vi "Start Sync.vi"(8 "error in (no error)":errorcluster, 11 "gRPC Server in":refnum<class "GreeterService.lvclass">) -> (0 "error out":errorcluster, 3 "gRPC Server out":refnum<class "GreeterService.lvclass">)   [LabVIEW 2019, in "Generated_server.lvlib" / "GreeterService.lvclass"]
uses:
  GreeterService.lvclass
  GreeterService.lvclass/GreeterService.ctl
  RPC Messages/Response.ctl
  RPC Messages/Response_response_oneof/Response_response_oneof.lvclass
  RPC Messages/Request_request_oneof/Request_request_oneof.lvclass/Request_request_oneof.ctl
  RPC Messages/Response_response_oneof/Response_response_oneof.lvclass/Response_response_oneof.ctl
  Generated_server.lvlib
  RPC Messages/Request_request_oneof/Request_request_oneof.lvclass
  <vilib>/gRPC/LabVIEW gRPC Library/grpc-lvsupport-release.lvlib
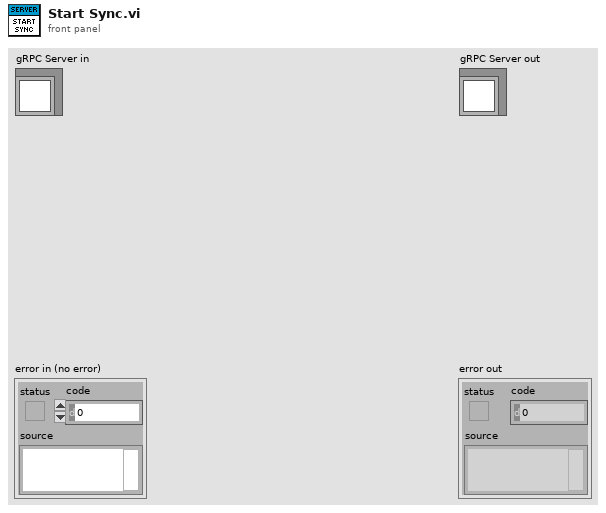
[diagram p1: front panel]
types:
  T1 = typedef "Generated_server.lvlib/Response.ctl" = cluster{"new_age":i32, "Response_response_oneof":refnum<class "Response_response_oneof.lvclass">}
  T2 = typedef "Generated_server.lvlib/GreeterService.lvclass/Server Internal UEs.ctl" = cluster{"GreeterService UnaryMethod Internal UE":refnum<user-event>, "GreeterService ServerStreamingMethod Internal UE":refnum<user-event>, "GreeterService ClientStreamingMethod Internal UE":refnum<user-event>, "GreeterService BidirectionalStreamingMethod Internal UE":refnum<user-event>}
  T3 = typedef "Generated_server.lvlib/GreeterService.lvclass/Server gRPC UEs.ctl" = cluster{"GreeterService UnaryMethod gRPC UE":refnum<user-event>, "GreeterService ServerStreamingMethod gRPC UE":refnum<user-event>, "GreeterService ClientStreamingMethod gRPC UE":refnum<user-event>, "GreeterService BidirectionalStreamingMethod gRPC UE":refnum<user-event>}
  T4 = typedef "grpc-lvsupport-release.lvlib/grpcId.ctl" = u64
  T5 = typedef "Generated_server.lvlib/Request.ctl" = cluster{"age":i32, "Request_request_oneof":refnum<class "Request_request_oneof.lvclass">}
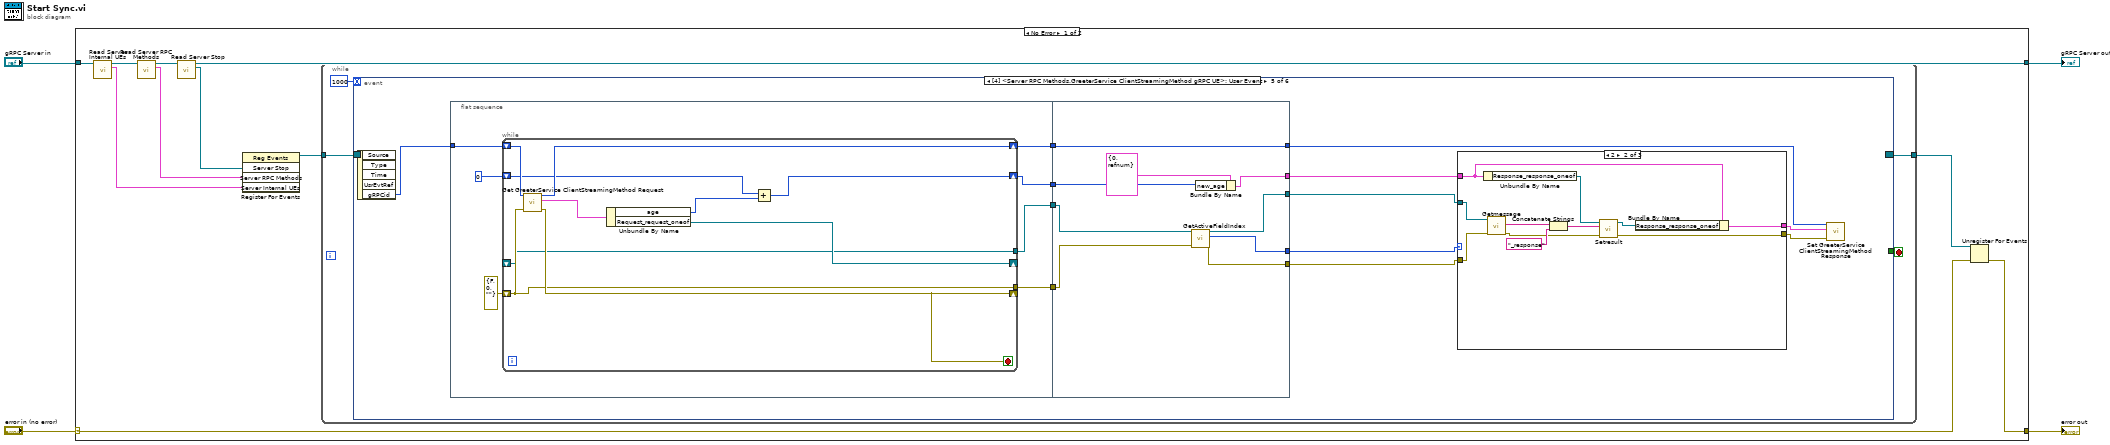
[diagram p0: block diagram]
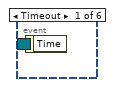
[diagram p2: hidden frame]
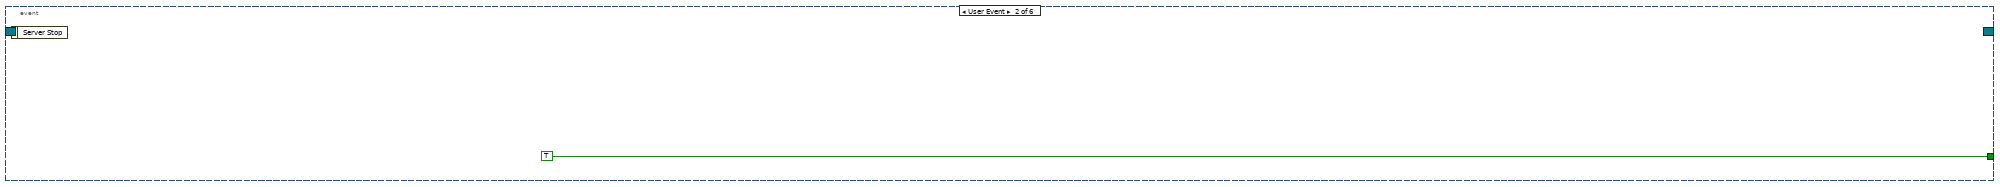
[diagram p3: hidden frame]
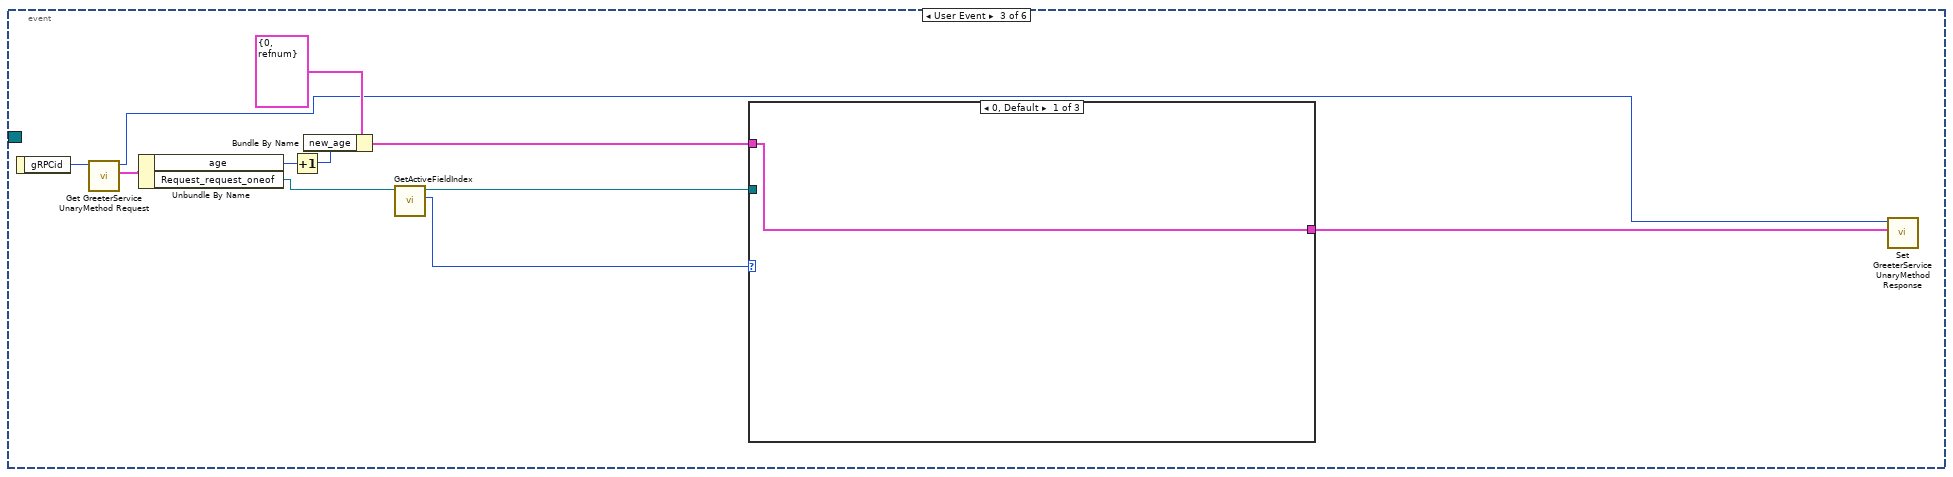
[diagram p4: hidden frame]
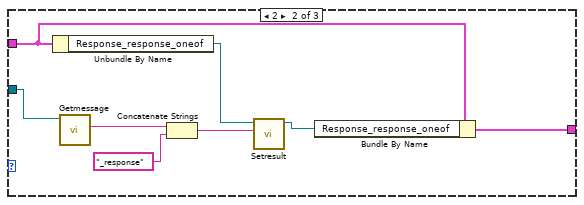
[diagram p5: hidden frame]
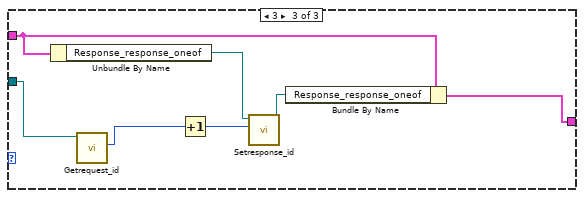
[diagram p6: hidden frame]
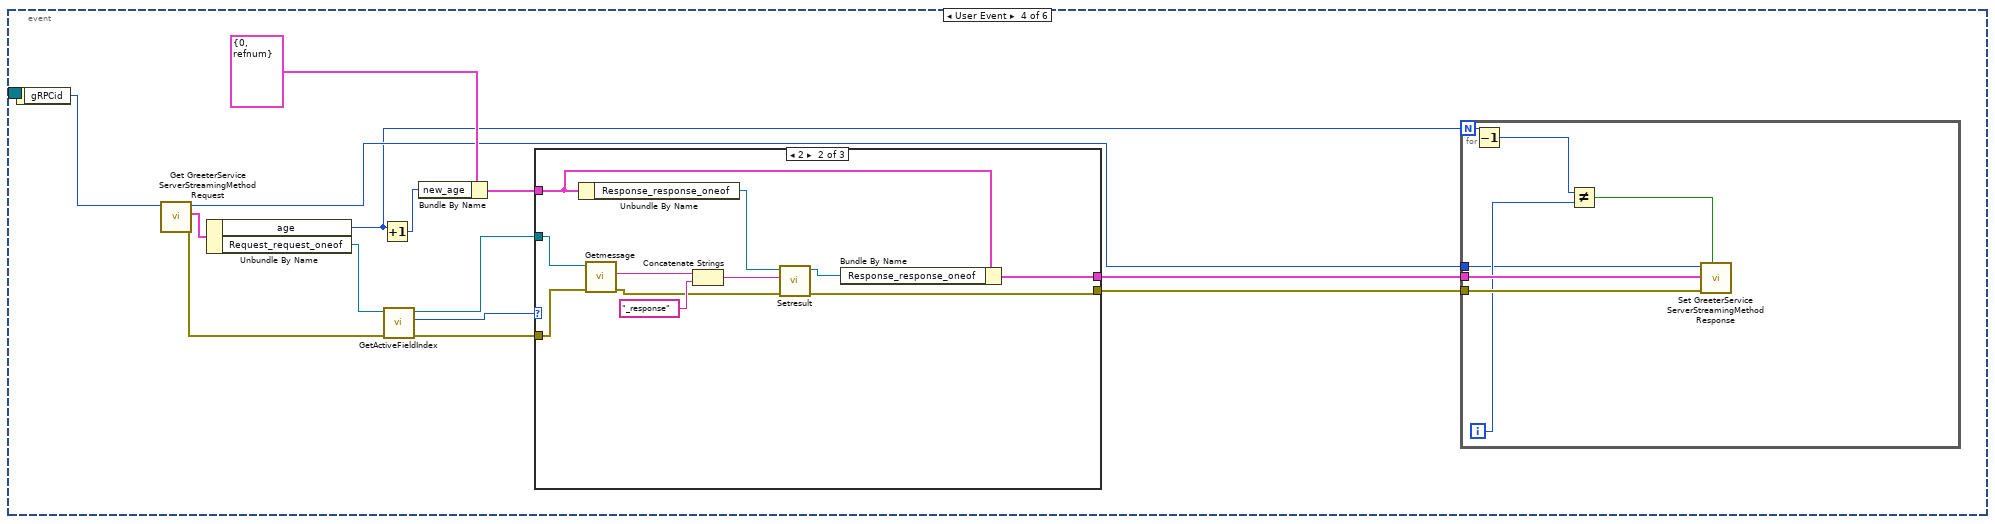
[diagram p7: hidden frame]
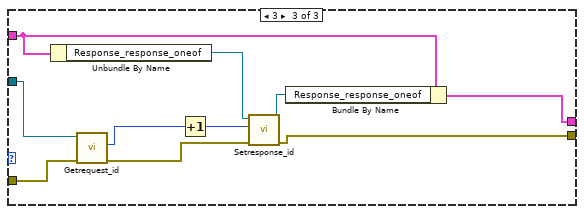
[diagram p9: hidden frame]
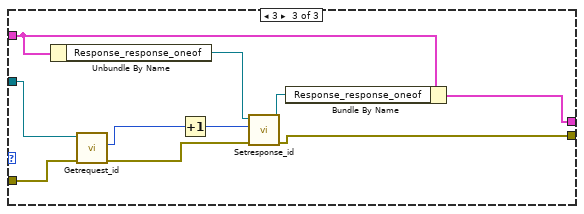
[diagram p11: hidden frame]
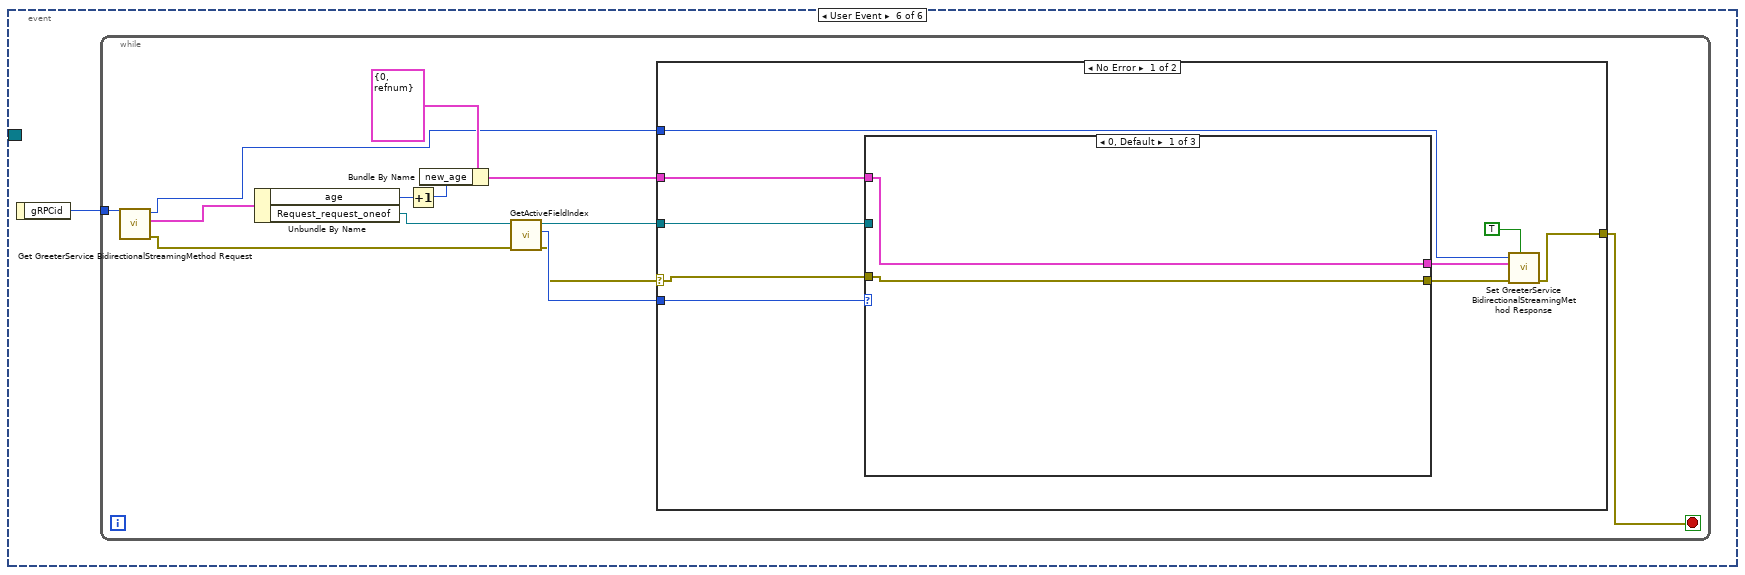
[diagram p12: hidden frame]
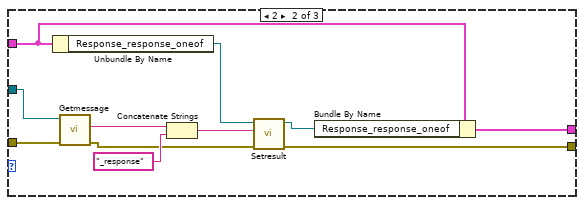
[diagram p13: hidden frame]
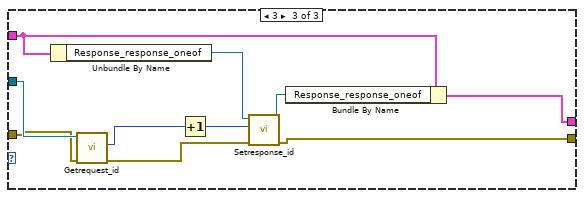
[diagram p14: hidden frame]
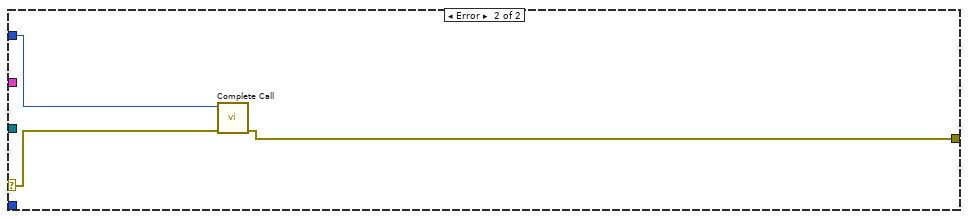
[diagram p15: hidden frame]
diagram:
  n1 = case shown="No Error" "error in (no error)" {
    selector: "error in (no error)" -> [w9 w203]
    tunnel: [w8 w203] -> w3
    tunnel: [w6 w202] -> w1
    tunnel: "gRPC Server in" -> [w15 w202]
    frame No Error {
      n2 = call "Read Server Internal UEs.vi"("SignalGeneratorService in"=w15) -> ("Server Internal UEs"=w13:T2, "SignalGeneratorService out"=w14:refnum<class "GreeterService.lvclass">)  [unwired: 8 in, 1 out]
      n3 = call "Read Server RPC Methods.vi"("SignalGeneratorService in"=w14) -> ("Server RPC Methods"=w7:T3, "SignalGeneratorService out"=w12:refnum<class "GreeterService.lvclass">)  [unwired: 8 in, 1 out]
      n4 = call-dynamic "Read Server Stop.vi"("iService in"=w12) -> ("Server Stop"=w5:refnum<user-event>, "iService out"=w6:refnum<class "GreeterService.lvclass">)  [unwired: 8 in, 1 out]
      n5 = register-events(w5, w7, w13) -> (reference out=w11:refnum<event-registration>)  [unwired: 2 in, 1 out]
      n6 = while {
        tunnel: w11 -> [w19]
        tunnel: [w17] -> w10
        stop <- w18 stop-if-true
        n7 = event "RPC Methods Event Structure" shown="[4] <Server RPC Methods.GreeterService ClientStreamingMethod gRPC UE>: User Event" {
          selector: w19 -> [_ _ _ _ _ _]
          dyn-events: [_ _ _ _ _ _] -> w17
          timeout: 1000 -> [_ _ _ _ _ _]
          tunnel: [_ TRUE _ _ _ _] -> w18
          event Timeout {
            n8 = event-data() -> ()  [unwired: 1 in, 1 out]
          }
          event User Event {
            n9 = event-data() -> ()  [unwired: 1 in, 1 out]
          }
          event User Event {
            n10 = event-data() -> ("gRPCid"=w31:T4)  [unwired: 1 in]
            n11 = call "Get GreeterService UnaryMethod Request.vi"("gRPCid"=w31) -> ("Message Data"=w30:T5, "gRPCid out"=w21:T4)  [unwired: 8 in, 1 out]
            n12 = Unbundle By Name(w30) -> ("age"=w27:i32, "Request_request_oneof"=w26:refnum<class "Request_request_oneof.lvclass">)
            n13 = Increment(x=w27) -> (x+1=w28:i32)
            n14 = Bundle By Name(cluster=T1 {"new_age"=0, "Response_response_oneof"=refnum} ("Response"), "new_age"=w28) -> (w23:T1)
            n15 = call "GetActiveFieldIndex.vi"("OneOfTemplate in"=w26) -> ("Active Field Index"=w25:i32, "OneOfTemplate out"=w24:refnum<class "Request_request_oneof.lvclass">)  [unwired: 8 in, 1 out]
            n16 = case shown="0, Default" w25 {
              tunnel: w24 -> [_ w40 w47]
              tunnel: w23 -> [w32 w35 w43]
              tunnel: [w32 w33 w41] -> w22
              frame 0, Default {
              }
              frame 2 {
                n17 = Unbundle By Name(w35) -> ("Response_response_oneof"=w36:refnum<class "Response_response_oneof.lvclass">)
                n18 = call "Getmessage.vi"("OneOfTemplate in"=w40) -> ("Get_Val"=w39:string)  [unwired: 8 in, 2 out]
                n19 = Concatenate Strings(w39, "_response") -> (w37:string)
                n20 = call "Setresult.vi"("Set_Val"=w37, "OneOfTemplate in"=w36) -> ("OneOfTemplate out"=w34:refnum<class "Response_response_oneof.lvclass">)  [unwired: 8 in, 1 out]
                n21 = Bundle By Name(cluster=w35, "Response_response_oneof"=w34) -> (w33:T1)
              }
              frame 3 {
                n22 = Unbundle By Name(w43) -> ("Response_response_oneof"=w44:refnum<class "Response_response_oneof.lvclass">)
                n23 = call "Getrequest_id.vi"("OneOfTemplate in"=w47) -> ("Get_Val"=w46:i32)  [unwired: 8 in, 2 out]
                n24 = Increment(x=w46) -> (x+1=w45:i32)
                n25 = call "Setresponse_id.vi"("Set_Val"=w45, "OneOfTemplate in"=w44) -> ("OneOfTemplate out"=w42:refnum<class "Response_response_oneof.lvclass">)  [unwired: 8 in, 1 out]
                n26 = Bundle By Name(cluster=w43, "Response_response_oneof"=w42) -> (w41:T1)
              }
            }
            n27 = call "Set GreeterService UnaryMethod Response.vi"("Message Data"=w22, "gRPCid in"=w21) -> ()  [unwired: 9 in, 1 out]
          }
          event User Event {
            n28 = event-data() -> ("gRPCid"=w61:T4)  [unwired: 1 in]
            n29 = call "Get GreeterService ServerStreamingMethod Request.vi"("gRPCid"=w61) -> ("error out"=w52:errorcluster, "Message Data"=w60:T5, "gRPCid out"=w49:T4)  [unwired: 8 in]
            n30 = Unbundle By Name(w60) -> ("age"=w48:i32, "Request_request_oneof"=w57:refnum<class "Request_request_oneof.lvclass">)
            n31 = Increment(x=w48) -> (x+1=w54:i32)
            n32 = call "GetActiveFieldIndex.vi"("error in (no error)"=w52, "OneOfTemplate in"=w57) -> ("error out"=w51:errorcluster, "Active Field Index"=w55:i32, "OneOfTemplate out"=w56:refnum<class "Request_request_oneof.lvclass">)  [unwired: 7 in]
            n33 = Bundle By Name(cluster=T1 {"new_age"=0, "Response_response_oneof"=refnum} ("Response"), "new_age"=w54) -> (w58:T1)
            n34 = case shown="2" w55 {
              tunnel: w56 -> [_ w74 w84]
              tunnel: w58 -> [w63 w69 w80]
              tunnel: [w63 w67 w78] -> w53
              tunnel: w51 -> [w62 w66 w77]
              tunnel: [w62 w64 w75] -> w50
              frame 0, Default {
              }
              frame 2 {
                n35 = Unbundle By Name(w69) -> ("Response_response_oneof"=w70:refnum<class "Response_response_oneof.lvclass">)
                n36 = call "Getmessage.vi"("error in (no error)"=w66, "OneOfTemplate in"=w74) -> ("error out"=w65:errorcluster, "Get_Val"=w73:string)  [unwired: 7 in, 1 out]
                n37 = Concatenate Strings(w73, "_response") -> (w71:string)
                n38 = call "Setresult.vi"("error in (no error)"=w65, "Set_Val"=w71, "OneOfTemplate in"=w70) -> ("error out"=w64:errorcluster, "OneOfTemplate out"=w68:refnum<class "Response_response_oneof.lvclass">)  [unwired: 7 in]
                n39 = Bundle By Name(cluster=w69, "Response_response_oneof"=w68) -> (w67:T1)
              }
              frame 3 {
                n40 = Unbundle By Name(w80) -> ("Response_response_oneof"=w81:refnum<class "Response_response_oneof.lvclass">)
                n41 = call "Getrequest_id.vi"("error in (no error)"=w77, "OneOfTemplate in"=w84) -> ("error out"=w76:errorcluster, "Get_Val"=w83:i32)  [unwired: 7 in, 1 out]
                n42 = Increment(x=w83) -> (x+1=w82:i32)
                n43 = call "Setresponse_id.vi"("error in (no error)"=w76, "Set_Val"=w82, "OneOfTemplate in"=w81) -> ("error out"=w75:errorcluster, "OneOfTemplate out"=w79:refnum<class "Response_response_oneof.lvclass">)  [unwired: 7 in]
                n44 = Bundle By Name(cluster=w80, "Response_response_oneof"=w79) -> (w78:T1)
              }
            }
            n45 = for {
              N: w48 -> [w86]
              tunnel: w53 -> [w91]
              tunnel: w50 -> [w90]
              tunnel: w49 -> [w87]
              i -> [w89]
              n46 = Decrement(x=w86) -> (x-1=w85:i32)
              n47 = Not Equal?(x=w85, y=w89) -> (x != y?=w88:bool)
              n48 = call "Set GreeterService ServerStreamingMethod Response.vi"("Streaming? (F)"=w88, "error in (no error)"=w90, "Message Data"=w91, "gRPCid in"=w87) -> ()  [unwired: 7 in, 1 out]
            }
          }
          event User Event {
            n49 = event-data() -> ("gRPCid"=w103:T4)  [unwired: 1 in, 4 out]
            n50 = flat-sequence {
              tunnel: w103 -> [w110]
              tunnel: [w108] -> w100
              tunnel: [w107] -> w99
              tunnel: [w106] -> w98
              tunnel: [w105] -> w97
              tunnel: [w129] -> w92
              tunnel: w100 -> [w125]
              tunnel: w99 -> [w129]
              tunnel: w98 -> [w128]
              tunnel: w97 -> [w127]
              tunnel: [w124] -> w96
              tunnel: [w123] -> w95
              tunnel: [w122] -> w94
              tunnel: [w121] -> w93
              frame #0 {
                n51 = while {
                  shift-right: [w115] -> w108
                  shift-left: 0 -> [w116]
                  shift-right: [w114] -> _
                  shift-left: _ -> [w111]
                  shift-right: [w118] -> w107
                  shift-left: w110 -> [w119]
                  shift-right: [w113] -> _
                  shift-left: errorcluster {"status"=FALSE, "code"=0, "source"=""} ("error out") -> [w112]
                  tunnel: [w112] -> w106
                  tunnel: [w111] -> w105
                  stop <- w113 stop-if-true
                  n52 = call "Get GreeterService ClientStreamingMethod Request.vi"("error in (no error)"=w112, "gRPCid"=w119) -> ("error out"=w113:errorcluster, "Message Data"=w120:T5, "gRPCid out"=w118:T4)  [unwired: 7 in]
                  n53 = Unbundle By Name(w120) -> ("age"=w117:i32, "Request_request_oneof"=w114:refnum<class "Request_request_oneof.lvclass">)
                  n54 = Add(x=w116, y=w117) -> (x+y=w115:i32)
                }
              }
              frame #1 {
                n55 = call "GetActiveFieldIndex.vi"("error in (no error)"=w128, "OneOfTemplate in"=w127) -> ("error out"=w124:errorcluster, "Active Field Index"=w123:i32, "OneOfTemplate out"=w122:refnum<class "Request_request_oneof.lvclass">)  [unwired: 7 in]
                n56 = Bundle By Name(cluster=T1 {"new_age"=0, "Response_response_oneof"=refnum} ("Response"), "new_age"=w125) -> (w121:T1)
              }
            }
            n57 = case shown="2" w95 {
              tunnel: w94 -> [_ w142 w152]
              tunnel: w93 -> [w131 w137 w148]
              tunnel: [w131 w135 w146] -> w102
              tunnel: w96 -> [w130 w134 w145]
              tunnel: [w130 w132 w143] -> w101
              frame 0, Default {
              }
              frame 2 {
                n58 = Unbundle By Name(w137) -> ("Response_response_oneof"=w138:refnum<class "Response_response_oneof.lvclass">)
                n59 = call "Getmessage.vi"("error in (no error)"=w134, "OneOfTemplate in"=w142) -> ("error out"=w133:errorcluster, "Get_Val"=w141:string)  [unwired: 7 in, 1 out]
                n60 = Concatenate Strings(w141, "_response") -> (w139:string)
                n61 = call "Setresult.vi"("error in (no error)"=w133, "Set_Val"=w139, "OneOfTemplate in"=w138) -> ("error out"=w132:errorcluster, "OneOfTemplate out"=w136:refnum<class "Response_response_oneof.lvclass">)  [unwired: 7 in]
                n62 = Bundle By Name(cluster=w137, "Response_response_oneof"=w136) -> (w135:T1)
              }
              frame 3 {
                n63 = Unbundle By Name(w148) -> ("Response_response_oneof"=w149:refnum<class "Response_response_oneof.lvclass">)
                n64 = call "Getrequest_id.vi"("error in (no error)"=w145, "OneOfTemplate in"=w152) -> ("error out"=w144:errorcluster, "Get_Val"=w151:i32)  [unwired: 7 in, 1 out]
                n65 = Increment(x=w151) -> (x+1=w150:i32)
                n66 = call "Setresponse_id.vi"("error in (no error)"=w144, "Set_Val"=w150, "OneOfTemplate in"=w149) -> ("error out"=w143:errorcluster, "OneOfTemplate out"=w147:refnum<class "Response_response_oneof.lvclass">)  [unwired: 7 in]
                n67 = Bundle By Name(cluster=w148, "Response_response_oneof"=w147) -> (w146:T1)
              }
            }
            n68 = call "Set GreeterService ClientStreamingMethod Response.vi"("error in (no error)"=w101, "Message Data"=w102, "gRPCid in"=w92) -> ()  [unwired: 8 in, 1 out]
          }
          event User Event {
            n69 = event-data() -> ("gRPCid"=w153:T4)  [unwired: 1 in]
            n70 = while {
              tunnel: w153 -> [w159]
              stop <- w154 stop-if-true
              n71 = call "Get GreeterService BidirectionalStreamingMethod Request.vi"("gRPCid"=w159) -> ("error out"=w156:errorcluster, "Message Data"=w157:T5, "gRPCid out"=w158:T4)  [unwired: 8 in]
              n72 = Unbundle By Name(w157) -> ("age"=w164:i32, "Request_request_oneof"=w163:refnum<class "Request_request_oneof.lvclass">)
              n73 = Increment(x=w164) -> (x+1=w165:i32)
              n74 = Bundle By Name(cluster=T1 {"new_age"=0, "Response_response_oneof"=refnum} ("Response"), "new_age"=w165) -> (w160:T1)
              n75 = call "GetActiveFieldIndex.vi"("error in (no error)"=w156, "OneOfTemplate in"=w163) -> ("error out"=w155:errorcluster, "Active Field Index"=w162:i32, "OneOfTemplate out"=w161:refnum<class "Request_request_oneof.lvclass">)  [unwired: 7 in]
              n76 = case shown="No Error" w155 {
                selector: w155 -> [w169 w200]
                tunnel: w162 -> [w175 _]
                tunnel: w161 -> [w174 _]
                tunnel: w160 -> [w173 _]
                tunnel: w158 -> [w172 w201]
                tunnel: [w167 w199] -> w154
                frame No Error {
                  n77 = case shown="0, Default" w175 {
                    tunnel: w174 -> [_ w188 w198]
                    tunnel: w173 -> [w177 w183 w194]
                    tunnel: [w177 w181 w192] -> w171
                    tunnel: w169 -> [w176 w180 w191]
                    tunnel: [w176 w178 w189] -> w168
                    frame 0, Default {
                    }
                    frame 2 {
                      n78 = Unbundle By Name(w183) -> ("Response_response_oneof"=w184:refnum<class "Response_response_oneof.lvclass">)
                      n79 = call "Getmessage.vi"("error in (no error)"=w180, "OneOfTemplate in"=w188) -> ("error out"=w179:errorcluster, "Get_Val"=w187:string)  [unwired: 7 in, 1 out]
                      n80 = Concatenate Strings(w187, "_response") -> (w185:string)
                      n81 = call "Setresult.vi"("error in (no error)"=w179, "Set_Val"=w185, "OneOfTemplate in"=w184) -> ("error out"=w178:errorcluster, "OneOfTemplate out"=w182:refnum<class "Response_response_oneof.lvclass">)  [unwired: 7 in]
                      n82 = Bundle By Name(cluster=w183, "Response_response_oneof"=w182) -> (w181:T1)
                    }
                    frame 3 {
                      n83 = Unbundle By Name(w194) -> ("Response_response_oneof"=w195:refnum<class "Response_response_oneof.lvclass">)
                      n84 = call "Getrequest_id.vi"("error in (no error)"=w191, "OneOfTemplate in"=w198) -> ("error out"=w190:errorcluster, "Get_Val"=w197:i32)  [unwired: 7 in, 1 out]
                      n85 = Increment(x=w197) -> (x+1=w196:i32)
                      n86 = call "Setresponse_id.vi"("error in (no error)"=w190, "Set_Val"=w196, "OneOfTemplate in"=w195) -> ("error out"=w189:errorcluster, "OneOfTemplate out"=w193:refnum<class "Response_response_oneof.lvclass">)  [unwired: 7 in]
                      n87 = Bundle By Name(cluster=w194, "Response_response_oneof"=w193) -> (w192:T1)
                    }
                  }
                  n88 = call "Set GreeterService BidirectionalStreamingMethod Response.vi"("Streaming? (F)"=TRUE, "error in (no error)"=w168, "Message Data"=w171, "gRPCid in"=w172) -> ("error out"=w167:errorcluster)  [unwired: 7 in]
                }
                frame Error {
                  n89 = call <vilib>:"Complete Call.vi"("gRPCid"=w201, "error in"=w200) -> ("error out"=w199:errorcluster)  [unwired: 8 in]
                }
              }
            }
          }
        }
      }
      n90 = Unregister For Events(event registration refnum=w10, error in=w9) -> (error out=w8:errorcluster)
    }
    frame Error {
    }
  }
  "error out" <- w3
  "gRPC Server out" <- w1
